vi "usrp get tx lo export enabled.vi"(7 "result_out":i32, 8 "error in (no error)":errorcluster, 9 "chan":u64, 10 "name":string, 11 "h":u64) -> (0 "error out":errorcluster, 3 "function return":u32(ring), 5 "result_out out":i32)   [LabVIEW 2023, in "uhd.lvlib"]
doc: "UHD_API uhd_error uhd_usrp_get_tx_lo_export_enabled(\n uhd_usrp_handle h, const char* name, size_t chan, bool* result_out);"
uses:
  <userlib>/uhd/uhd.lvlib
  <userlib>/uhd/uhd.dll
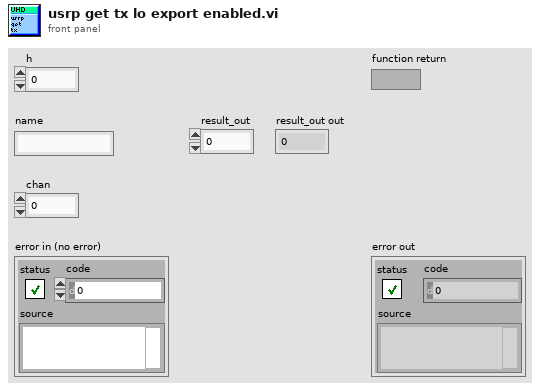
[diagram p1: front panel]
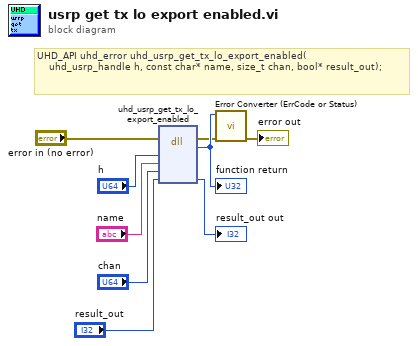
[diagram p0: block diagram]
diagram:
  # "UHD_API uhd_error uhd_usrp_get_tx_lo_export_enabled(\n    uhd_usrp_handle h, const char* name, size_t chan, bool* result_out);"
  n1 = dll-call lib="C:/Program Files/National Instruments/LabVIEW 2023/user.lib/uhd/uhd.*" fn="uhd_usrp_get_tx_lo_export_enabled"(error in="error in (no error)", "h"="h", "name"="name", "chan"="chan", "result_out"="result_out") -> (error out=w2:errorcluster, w9:u32, "result_out"=→"result_out out":i32)  [unwired: 5 in, 1 out]
  "function return" <- w9
  n2 = call <userlib>:"Error Converter (ErrCode or Status).vi"("error in (no error)"=w2, "error code"=w9) -> ("error out"=→"error out":errorcluster)  [unwired: 9 in]
